vi "Write Data To File.vi"(5 "file path (use dialog)":path=path "random_generated_data.txt", 7 "Array":dbl[][](array[numeric]), 9 "error in":errorcluster) -> (8 "error out":errorcluster)   [LabVIEW 2014]
uses:
  <vilib>/Utility/file.llb/Write To Spreadsheet File (DBL).vi
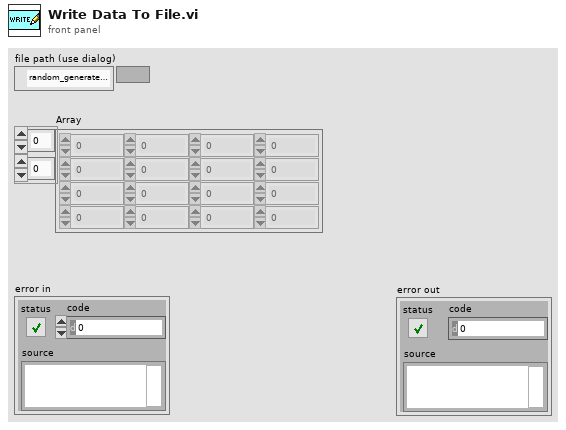
[diagram p1: front panel]
types:
  T1 = enum16{"open", "replace", "create", "open or create", "replace or create", "replace or create with confirmation"}
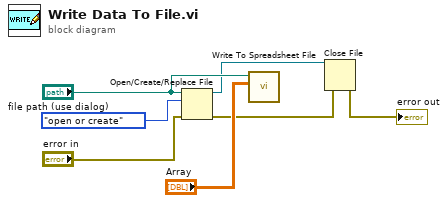
[diagram p0: block diagram]
diagram:
  n1 = Open/Create/Replace File(file path (use dialog)="file path (use dialog)", error in="error in", operation (0:open)=T1."open or create") -> (refnum out=w2:refnum<file>, error out=w1:errorcluster)  [unwired: 3 in, 1 out]
  n2 = call-poly <vilib>:"Write To Spreadsheet File.vi"("2D data"="Array", "file path (dialog if empty)"="file path (use dialog)") -> ()  [unwired: 6 in, 1 out]
  n3 = Close File(refnum=w2, error in=w1) -> (error out=→"error out":errorcluster)  [unwired: 1 out]
